vi "Tree_GetTag FromIndex.vi"(8 "Error In":errorcluster, 10 "Index IN":i32, 11 "Tree Refnum IN":refnum<vi>) -> (0 "Error Out":errorcluster, 2 "Tag OUT":string, 3 "Tree Refnum OUT":refnum<vi>)   [LabVIEW 2012]
doc: "SciScan 1.2 160622"
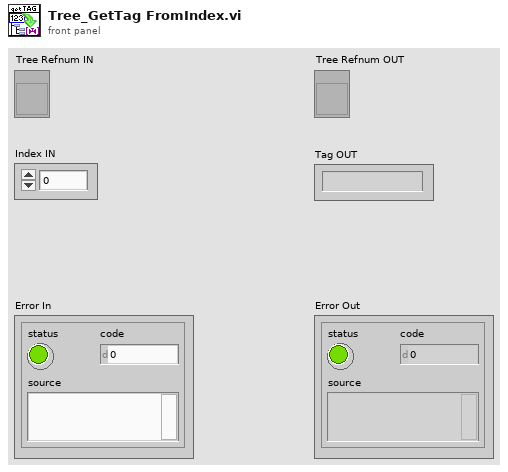
[diagram p1: front panel]
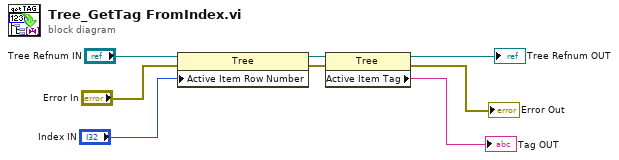
[diagram p0: block diagram]
diagram:
  n1 = property class="Tree"(reference="Tree Refnum IN", error in="Error In", "Active Item Row Number"="Index IN") -> (reference out=w7:refnum<vi>, error out=w6:errorcluster)
  n2 = property class="Tree"(reference=w7, error in=w6) -> (reference out=→"Tree Refnum OUT":refnum<vi>, error out=→"Error Out":errorcluster, "Active Item Tag"=→"Tag OUT":string)
